vi "Append Port To Source Host.vi"(0 "message in":T1, 5 "source port":u16, 11 "error in":errorcluster) -> (4 "message out":T1, 15 "error out":errorcluster)   [LabVIEW 2012, in "Car Wash.lvlib" / "AMC.lvlib"]
uses:
  AMC.lvlib
  Message.ctl
  Tools/Keyed Array/KeyedArray.ctl
  Tools/Keyed Array/Tools_KeyedArray.lvlib
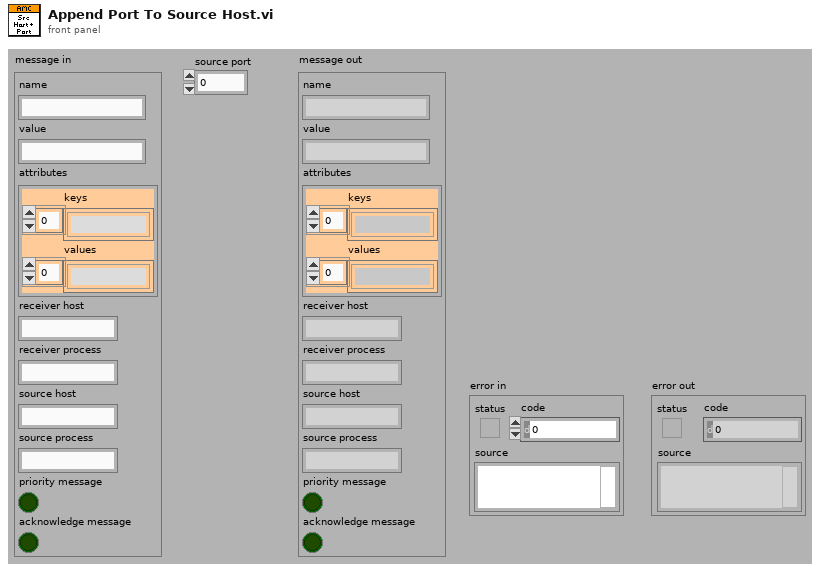
[diagram p1: front panel]
types:
  T1 = typedef "Car Wash.lvlib/AMC.lvlib/Message.ctl" = cluster{"name":string, "value":string, "attributes":T2, "receiver host":string, "receiver process":string, "source host":string, "source process":string, "priority message":bool, "acknowledge message":bool}
  T2 = typedef "Car Wash.lvlib/Tools_KeyedArray.lvlib/KeyedArray.ctl" = cluster{"keys":string[], "values":string[]}
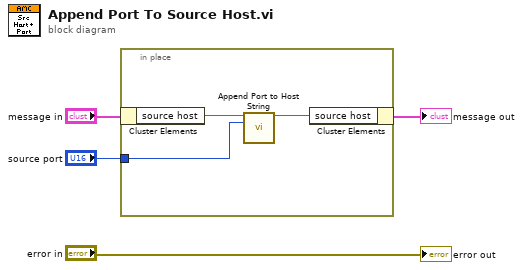
[diagram p0: block diagram]
diagram:
  n1 = in-place {
    in-place-border: "source port" -> [w5]
    n2 = in-place-cluster #1("message in") -> ("source host"=w7:string)
    n3 = call "Append Port to Host String.vi"("host in"=w7, "port"=w5) -> ("host out"=w6:string)  [unwired: 13 in]
    n4 = in-place-cluster #1("source host"=w6) -> (→"message out":T1)
  }
  "error out" <- "error in"
